vi "String Length in Runes.vi"(8 "error in (no error)":errorcluster, 11 "UTF8 in":refnum<class "UTF-8 String.lvclass">) -> (0 "error out":errorcluster, 2 "Length":i32, 3 "UTF8 out":refnum<class "UTF-8 String.lvclass">)   [LabVIEW 2019, in "JKI Unicode.lvlib" / "UTF-8 String.lvclass"]
doc: "JKI Unicode 1.0.0.7\nTomi Maila - JKI\nCopyright (c) 2016, JKI"
uses:
  UTF-8 String.lvclass
  UTF-8 String.lvclass/UTF-8 String.ctl
  Bytes In Rune.vi
  <vilib>/Utility/error.llb/Error Cluster From Error Code.vi
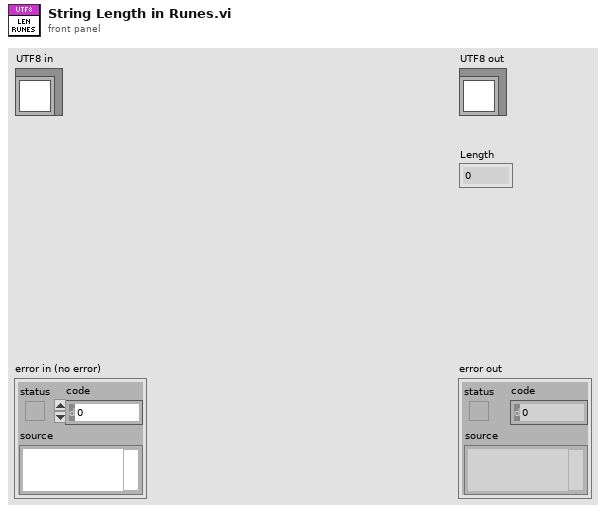
[diagram p1: front panel]
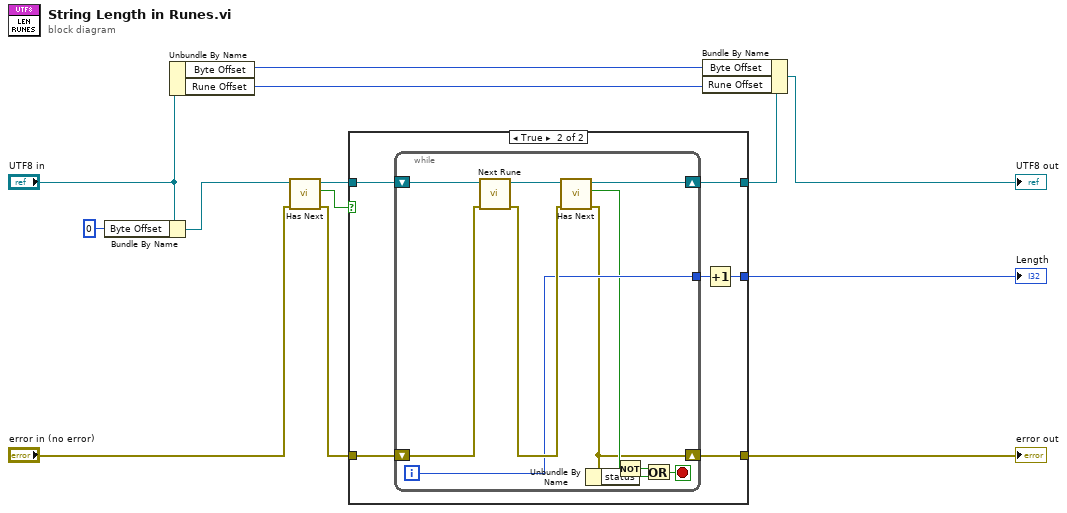
[diagram p0: block diagram]
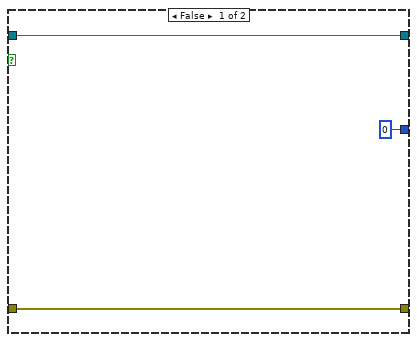
[diagram p2: hidden frame]
diagram:
  n1 = Bundle By Name(cluster="UTF8 in", "Byte Offset"=0) -> (w6:refnum<class "UTF-8 String.lvclass">)
  n2 = Unbundle By Name("UTF8 in") -> ("Byte Offset"=w9:i32, "Rune Offset"=w8:i32)
  n3 = call "Has Next.vi"("error in (no error)"="error in (no error)", "UTF8 in"=w6) -> ("error out"=w2:errorcluster, "Has Next?"=w1:bool, "UTF8 out"=w4:refnum<class "UTF-8 String.lvclass">)  [unwired: 7 in]
  n4 = case shown="True" w1 {
    tunnel: [w14 w18] -> w13
    tunnel: [0 ("Rune") w17] -> w12
    tunnel: [w16 w19] -> w11
    tunnel: w4 -> [w16 w21]
    tunnel: w2 -> [w14 w20]
    frame False {
    }
    frame True {
      n5 = while {
        tunnel: [w28] -> w22
        shift-right: [w30] -> w19
        shift-left: w21 -> [w32]
        shift-right: [w24] -> w18
        shift-left: w20 -> [w31]
        i -> [w28]
        stop <- w26 stop-if-true
        n6 = call "Next Rune.vi"("error in (no error)"=w31, "UTF8 in"=w32) -> ("error out"=w29:errorcluster, "UTF8 out"=w33:refnum<class "UTF-8 String.lvclass">)  [unwired: 7 in, 1 out]
        n7 = call "Has Next.vi"("error in (no error)"=w29, "UTF8 in"=w33) -> ("error out"=w24:errorcluster, "Has Next?"=w27:bool, "UTF8 out"=w30:refnum<class "UTF-8 String.lvclass">)  [unwired: 7 in]
        n8 = Unbundle By Name(w24) -> ("status"=w23:bool)
        n9 = Not(x=w27) -> (.not. x?=w25:bool)
        n10 = Or(x=w25, y=w23) -> (x .or. y?=w26:bool)
      }
      n11 = Increment(x=w22) -> (x+1=w17:i32)
    }
  }
  "error out" <- w13
  "Length" <- w12
  n12 = Bundle By Name(cluster=w11, "Byte Offset"=w9, "Rune Offset"=w8) -> (→"UTF8 out":refnum<class "UTF-8 String.lvclass">)
